vi "Method.vi"(4 "Input B":refnum<class "Abs_Numeric.lvclass">, 5 "Input A":refnum<class "Abs_Time.lvclass">) -> (1 "Result":refnum<class "Abs_Time.lvclass">)   [LabVIEW 2021, in "Add_Time.lvclass"]
uses:
  Add_Time.lvclass
  Abs_Types/Time/Abs_Time.lvclass
  Abs_Types/Numeric/Abs_Numeric.lvclass
  C:/TSA/LV_Abstract/Source/Functions/Support/Function/Two Terminal/Time/AbsFunc_Two Term_Time.lvclass
  C:/Program Files (x86)/National Instruments/LabVIEW 2021/vi.lib/TSA/Abstract Data Classes/Abs_Types/Time/Abs_Time.lvclass
  Support/Function/Two Terminal/Time/AbsFunc_Two Term_Time.lvclass/AbsFunc_Two Term_Time.ctl
  Support/Function/Two Terminal/Time/Properties/Write Numeric A.vi
  Support/Function/Two Terminal/Time/Properties/Write Numeric B.vi
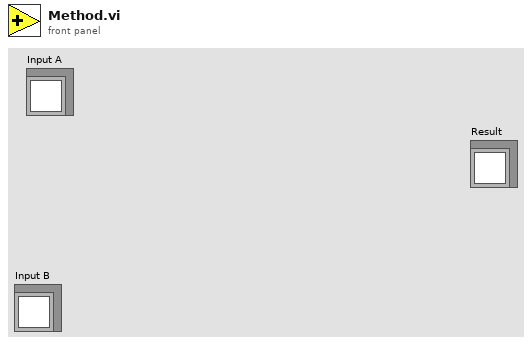
[diagram p1: front panel]
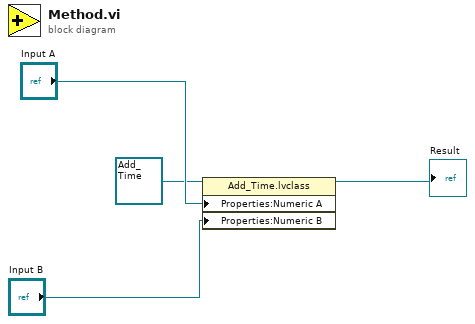
[diagram p0: block diagram]
diagram:
  n1 = property class="Add_Time.lvclass"(reference=refnum<class "Add_Time.lvclass"> refnum ("Functions.lvlib:Numeric.lvlib:Add_DBL.lvclass"), "Properties:Numeric A"="Input A", "Properties:Numeric B"="Input B") -> (reference out=→"Result":refnum<class "Add_Time.lvclass">)  [unwired: 1 in, 1 out]
